vi "04_Aug_By_Scale_Shift_Hue_By_Img.vi"() -> ()   [LabVIEW 2020]
uses:
  <vilib>/vision/NI_Vision_Development_Module.lvlib
panel:
  out "Progress":i32=859
  out "Total":i32=860
  in  "Image Type":T1=4 items=["Grayscale (U8)", "Grayscale (I16)", "Grayscale (SGL)", "Complex (CSG)", "RGB (U32)", "HSL (U32)", "RGB (U64)", "Grayscale (U16)"]
  in  "Scale":sgl=0.1 min=0 max=1 format="%#_2g"
  in  "Image Path (Destination)":path=path "D:/DNN/_AD/_from_Customers/2025_04_11_NIConnect_PCB5/1_Dataset/11_Augx4_Hue/Train/good"
  in  "Image Path (Source)":path=path "D:/DNN/_AD/_from_Customers/2025_04_11_NIConnect_PCB5/1_Dataset/11_Augx4_Hue/Train/good"
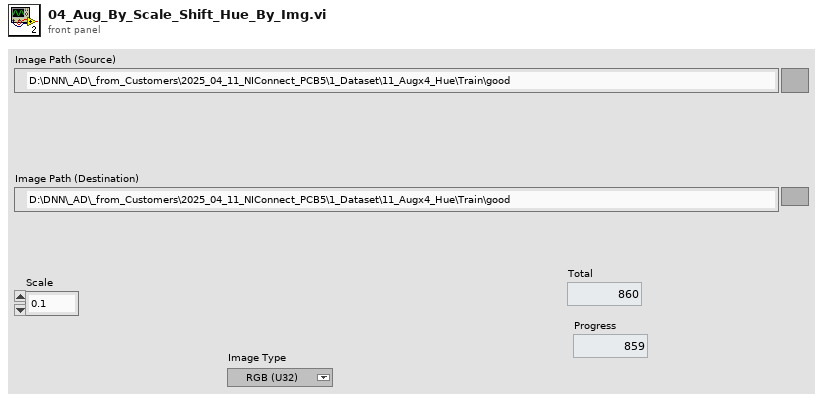
[diagram p1: front panel]
types:
  T1 = typedef "Image Type" = u32
  T2 = typedef "IMAQ Image.ctl" = refnum<image>
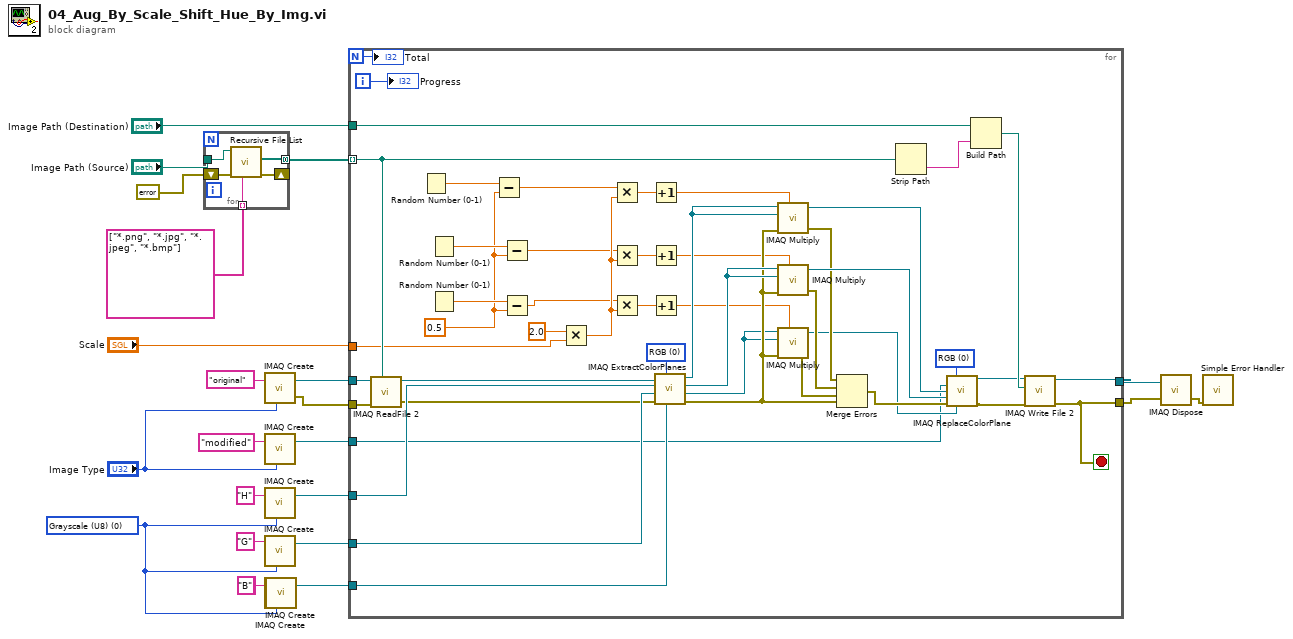
[diagram p0: block diagram]
diagram:
  w3 = T1 0 items=["Grayscale (U8)", "Grayscale (I16)", "Grayscale (SGL)", "Complex (CSG)", "RGB (U32)", "HSL (U32)", "RGB (U64)", "Grayscale (U16)"] ("Image Type")
  n1 = for {
    tunnel: "Image Path (Source)" -> [w28]
    tunnel: string[] ["*.png", "*.jpg", "*.jpeg", "*.bmp"] ("pattern") -> [w27] mode=indexing
    tunnel: [w26] -> w6 mode=concatenating
    shift-right: [w24] -> _
    shift-left: errorcluster {"status"=FALSE, "code"=0, "source"=""} ("error in (no error)") -> [w25]
    n2 = call <vilib>:"Recursive File List.vi"("pattern"=w27, "error in (no error)"=w25, "Folder Path"=w28) -> ("error out"=w24:errorcluster, "All Files in Dir"=w26:path[])  [unwired: 4 in, 3 out]
  }
  n3 = call "IMAQ Create"("Image Name"="original", "Image Type"="Image Type") -> ("New Image"=w22:T2, "error out"=w2:errorcluster)  [unwired: 3 in]
  n4 = call "IMAQ Create"("Image Name"="modified", "Image Type"="Image Type") -> ("New Image"=w16:T2)  [unwired: 3 in, 1 out]
  n5 = call "IMAQ Create"("Image Name"="H", "Image Type"=w3) -> ("New Image"=w14:T2)  [unwired: 3 in, 1 out]
  n6 = call "IMAQ Create"("Image Name"="G", "Image Type"=w3) -> ("New Image"=w11:T2)  [unwired: 3 in, 1 out]
  n7 = call "IMAQ Create"("Image Name"="B", "Image Type"=w3) -> ("New Image"=w10:T2)  [unwired: 3 in, 1 out]
  n8 = call "IMAQ Create"("Image Name"="B") -> ()  [unwired: 4 in, 2 out]
  n9 = for {
    N -> [w68]
    tunnel: w22 -> [w75]
    tunnel: "Image Path (Destination)" -> [w72]
    tunnel: [w73] -> w21
    tunnel: "Scale" -> [w30]
    tunnel: w16 -> [w29]
    tunnel: [w74] -> w20
    tunnel: w14 -> [w35]
    tunnel: w11 -> [w34]
    tunnel: w10 -> [w33]
    tunnel: w6 -> [w70] mode=indexing
    tunnel: w2 -> [w31]
    i -> [w67]
    stop <- w74 stop-if-true
    w44 = 0.5 ("y")
    w65 = u16 0 items=["RGB", "HSL", "HSV", "HSI"] ("Color Mode")
    w66 = u16 0 items=["RGB", "HSL", "HSV", "HSI"] ("Color Mode")
    n10 = call "IMAQ ReadFile 2"("File Path"=w70, "error in (no error)"=w31, "Image"=w75) -> ("error out"=w32:errorcluster, "Image Out"=w36:T2)  [unwired: 4 in, 3 out]
    n11 = Random Number (0-1)() -> (number: 0 to 1=w61:dbl)
    n12 = Random Number (0-1)() -> (number: 0 to 1=w63:dbl)
    n13 = Random Number (0-1)() -> (number: 0 to 1=w62:dbl)
    n14 = Subtract(x=w61, y=w44) -> (x-y=w45:dbl)
    n15 = Subtract(x=w63, y=w44) -> (x-y=w46:dbl)
    n16 = Subtract(x=w62, y=w44) -> (x-y=w47:dbl)
    n17 = Multiply(x=2.0 ("y"), y=w30) -> (x*y=w49:dbl)
    n18 = Multiply(x=w45, y=w49) -> (x*y=w50:dbl)
    n19 = Multiply(x=w46, y=w49) -> (x*y=w42:dbl)
    n20 = Multiply(x=w47, y=w49) -> (x*y=w43:dbl)
    n21 = Increment(x=w50) -> (x+1=w41:dbl)
    n22 = Increment(x=w42) -> (x+1=w40:dbl)
    n23 = Increment(x=w43) -> (x+1=w39:dbl)
    n24 = call "IMAQ ExtractColorPlanes"("Blue or Luma or Val or Inten Plane"=w33, "Color Mode"=w66, "error in (no error)"=w32, "Green or Sat Plane"=w34, "Red or Hue Plane"=w35, "Image Src"=w36) -> ("error out"=w53:errorcluster, "Blue or Luma or Val or Inten Plane out"=w52:T2, "Green or Sat Plane out"=w64:T2, "Red or Hue Plane out"=w60:T2)  [unwired: 2 in]
    n25 = call "IMAQ Multiply"("Image Src A"=w60, "Constant"=w41, "Image Dst"=w60, "error in (no error)"=w53) -> ("Image Dst Out"=w59:T2, "error out"=w56:errorcluster)  [unwired: 3 in]
    n26 = call "IMAQ Multiply"("Image Src A"=w64, "Constant"=w40, "Image Dst"=w64, "error in (no error)"=w53) -> ("Image Dst Out"=w58:T2, "error out"=w55:errorcluster)  [unwired: 3 in]
    n27 = call "IMAQ Multiply"("Image Src A"=w52, "Constant"=w39, "Image Dst"=w52, "error in (no error)"=w53) -> ("Image Dst Out"=w51:T2, "error out"=w54:errorcluster)  [unwired: 3 in]
    n28 = Merge Errors(w56, w55, w54, w53) -> (w57:errorcluster)
    n29 = Strip Path(path=w70) -> (name=w69:string)  [unwired: 1 out]
    n30 = call "IMAQ ReplaceColorPlane"("Color Mode"=w65, "Image Dst"=w29, "Red or Hue Plane"=w59, "Green or Sat Plane"=w58, "error in (no error)"=w57, "Blue or Luma or Val or Inten Plane"=w51) -> ("Image Dst Out"=w38:T2, "error out"=w37:errorcluster)  [unwired: 8 in]
    n31 = Build Path(base path=w72, name or relative path=w69) -> (appended path=w71:path)
    n32 = call-poly "IMAQ Write File 2"("error in (no error)"=w37, "File Path"=w71, "Image"=w38) -> ("error out"=w74:errorcluster, "Image Out (duplicate)"=w73:T2)  [unwired: 7 in]
    "Total" <- w68
    "Progress" <- w67
  }
  n33 = call "IMAQ Dispose"("Image"=w21, "error in (no error)"=w20) -> ("error out"=w19:errorcluster)  [unwired: 4 in]
  n34 = call <vilib>:"Simple Error Handler.vi"("error in (no error)"=w19) -> ()  [unwired: 4 in, 5 out]
